vi "Home.vi"(8 "error in (no error)":errorcluster, 11 "Stage_MadCityLabMicro in":refnum<class "Stage_MadCityLabMicro.lvclass">) -> (0 "error out":errorcluster, 3 "Stage_MadCityLabMicro out":refnum<class "Stage_MadCityLabMicro.lvclass">)   [LabVIEW 2020, in "Stage_MadCityLabMicro.lvlib" / "Stage_MadCityLabMicro.lvclass"]
uses:
  Stage_MadCityLabMicro.lvclass
  Stage_MadCityLabMicro.lvclass/Stage_MadCityLabMicro.ctl
  HAL Layer/Component/Stage/Stage/Stage.lvclass
  Dependency/MicroDrive.dll
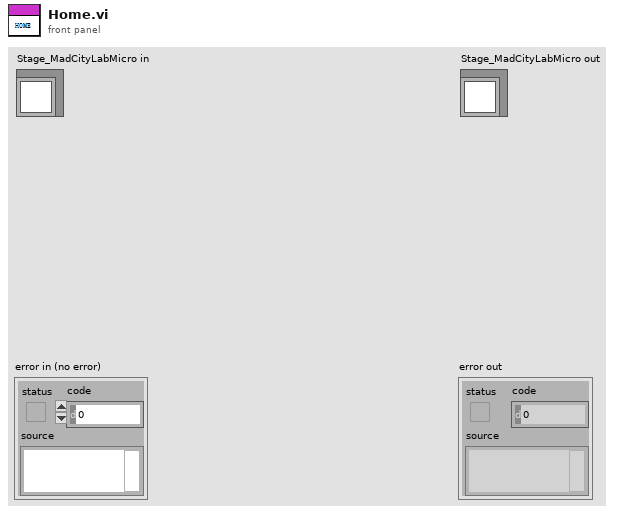
[diagram p1: front panel]
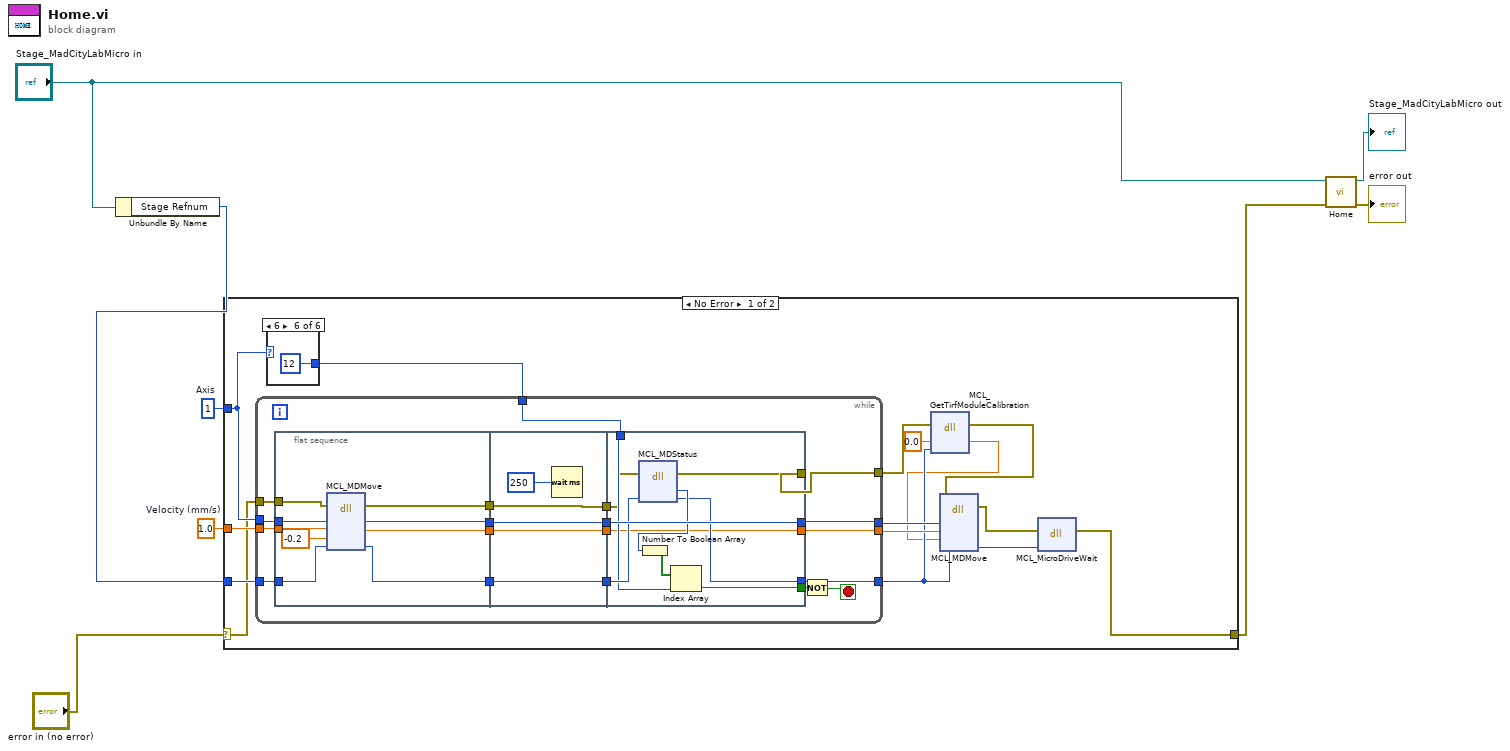
[diagram p0: block diagram]
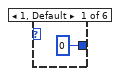
[diagram p2: hidden frame]
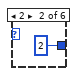
[diagram p3: hidden frame]
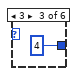
[diagram p4: hidden frame]
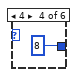
[diagram p5: hidden frame]
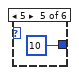
[diagram p6: hidden frame]
diagram:
  w3 = 1.0  # Velocity (mm/s)
  w4 = u16 1  # Axis
  n1 = Unbundle By Name("Stage_MadCityLabMicro in") -> ("Stage Refnum"=w5:i32)
  n2 = case shown="No Error" "error in (no error)" {
    selector: "error in (no error)" -> [w13 w73]
    tunnel: w3 -> [w23 _]
    tunnel: w5 -> [w22 _]
    tunnel: w4 -> [w19 _]
    tunnel: [w9 w73] -> w1
    frame No Error {
      n3 = case shown="6" w19 {
        tunnel: [0 2 4 8 10 12] -> w18
        frame 1, Default {
        }
        frame 2 {
        }
        frame 3 {
        }
        frame 4 {
        }
        frame 5 {
        }
        frame 6 {
        }
      }
      n4 = while {
        tunnel: w23 -> [w48]
        tunnel: w22 -> [w44]
        tunnel: [w43] -> w15
        tunnel: w19 -> [w46]
        tunnel: [w45] -> w21
        tunnel: w18 -> [w38]
        tunnel: [w34] -> w17
        tunnel: w13 -> [w33]
        tunnel: [w30] -> w12
        stop <- w47 stop-if-true
        n5 = flat-sequence {
          tunnel: w48 -> [w57]
          tunnel: w46 -> [w55]
          tunnel: w44 -> [w53]
          tunnel: [w54] -> w42
          tunnel: [w52] -> w41
          tunnel: [w51] -> w36
          tunnel: w33 -> [w50]
          tunnel: [w49] -> w32
          tunnel: w42 -> [w62]
          tunnel: w41 -> [w61]
          tunnel: [w62] -> w40
          tunnel: [w61] -> w39
          tunnel: w36 -> [w59]
          tunnel: [w59] -> w35
          tunnel: w32 -> [w58]
          tunnel: [w58] -> w31
          tunnel: [w68] -> w43
          tunnel: [w72] -> w45
          tunnel: w40 -> [w72]
          tunnel: w39 -> [w69]
          tunnel: w38 -> [w67]
          tunnel: [w66] -> w37
          tunnel: w35 -> [w65]
          tunnel: [w65] -> w34
          tunnel: w31 -> [w64]
          tunnel: [w63] -> w30
          frame #0 {
            n6 = dll-call lib="E:/Development/DevHardSoftware/MMicroscopyAF/Model/Real Hardware/Stage_MadCityLabMicro/Stage_MadCityLabMicro/Dependency/MicroDrive.dll" fn="MCL_MDMove"(error in=w50, "axis"=w55, "velocity"=w57, "distance"=-0.2, "handle"=w53) -> (error out=w49:errorcluster, "axis"=w54:i32, "velocity"=w51:dbl, "handle"=w52:i32)  [unwired: 3 in, 2 out]
          }
          frame #1 {
            n7 = Wait (ms)(milliseconds to wait=u32 250) -> ()  [unwired: 1 out]
          }
          frame #2 {
            n8 = dll-call lib="E:/Development/DevHardSoftware/MMicroscopyAF/Model/Real Hardware/Stage_MadCityLabMicro/Stage_MadCityLabMicro/Dependency/MicroDrive.dll" fn="MCL_MDStatus"(error in=w64, "handle"=w69) -> (error out=w63:errorcluster, "status"=w71:u16, "handle"=w68:i32)  [unwired: 2 in, 3 out]
            n9 = Number To Boolean Array(number=w71) -> (Boolean array=w70:bool[])
            n10 = Index Array(array=w70, index=w67) -> (element=w66:bool)
          }
        }
        n11 = Not(x=w37) -> (.not. x?=w47:bool)
      }
      n12 = dll-call lib="E:/Development/DevHardSoftware/MMicroscopyAF/Model/Real Hardware/Stage_MadCityLabMicro/Stage_MadCityLabMicro/Dependency/MicroDrive.dll" fn="MCL_GetTirfModuleCalibration"(error in=w12, "calMM"=0.0 ("distance"), "handle"=w15) -> (error out=w11:errorcluster, "calMM"=w14:dbl)  [unwired: 3 in, 2 out]
      n13 = dll-call lib="E:/Development/DevHardSoftware/MMicroscopyAF/Model/Real Hardware/Stage_MadCityLabMicro/Stage_MadCityLabMicro/Dependency/MicroDrive.dll" fn="MCL_MDMove"(error in=w11, "axis"=w21, "velocity"=w17, "distance"=w14, "handle"=w15) -> (error out=w10:errorcluster, "handle"=w20:i32)  [unwired: 4 in, 3 out]
      n14 = dll-call lib="E:/Development/DevHardSoftware/MMicroscopyAF/Model/Real Hardware/Stage_MadCityLabMicro/Stage_MadCityLabMicro/Dependency/MicroDrive.dll" fn="MCL_MicroDriveWait"(error in=w10, "handle"=w20) -> (error out=w9:errorcluster)  [unwired: 3 in, 2 out]
    }
    frame Error {
    }
  }
  n15 = call-parent "Home.vi"("error in (no error)"=w1, "Stage in"="Stage_MadCityLabMicro in") -> ("error out"=→"error out":errorcluster, "Stage out"=→"Stage_MadCityLabMicro out":refnum<class "Stage_MadCityLabMicro.lvclass">)  [unwired: 8 in]
